vi "人脸检测.vi"(8 "错误输入（无错误）":errorcluster, 9 "face Parameter":T1, 10 "access_token":string, 11 "client_in":T2) -> (0 "错误输出":errorcluster, 2 "body":string caption="体部", 3 "client_out":T2)   [LabVIEW 2025, in "Baidu api.lvlib"]
uses:
  Baidu api.lvlib
  <vilib>/httpClient/ClientHandle.ctl
  <vilib>/httpClient/POSTBuffer.vi
  <vilib>/httpClient/LabVIEWHTTPClient.lvlib
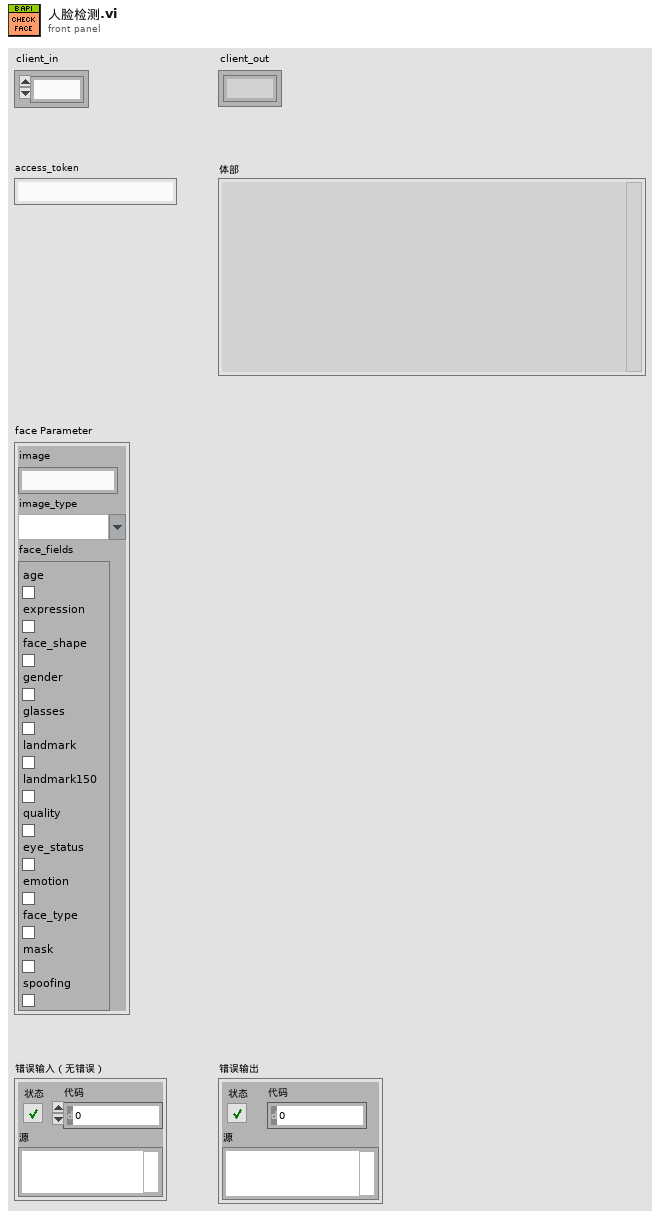
[diagram p1: front panel]
types:
  T1 = cluster{"image":string, "image_type":string, "face_fields ":cluster{"age":bool, "expression":bool, "face_shape":bool, "gender":bool, "glasses":bool, "landmark":bool, "landmark150":bool, "quality":bool, "eye_status":bool, "emotion":bool, "face_type":bool, "mask":bool, "spoofing":bool}}
  T2 = typedef "LabVIEWHTTPClient.lvlib/ClientHandle.ctl" = refnum<k1>
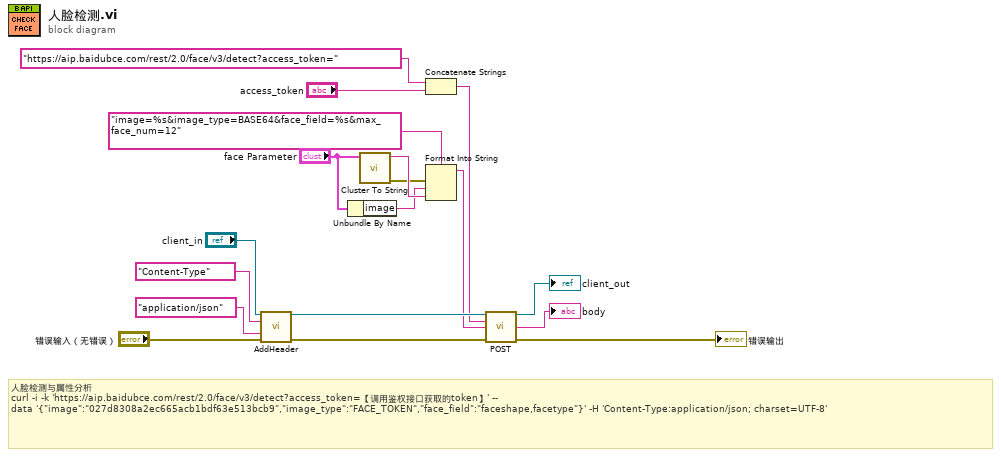
[diagram p0: block diagram]
diagram:
  # "人脸检测与属性分析\ncurl -i -k 'https://aip.baidubce.com/rest/2.0/face/v3/detect?access_token=【调用鉴权接口获取的token】' --\ndata '{\"image\":\"027d8308a2ec665acb1bdf63e513bcb9\",\"image_type\":\"FACE_TOKEN\",\"face_field\":\"faceshape,facetype\"}' -H 'Content-Type:application/json; charset=UTF-8'"
  n1 = call <vilib>:"AddHeader.vi"("client handle"="client_in", "header"="Content-Type", "value"="application/json", "error in (no error)"="错误输入（无错误）") -> ("client handle out"=w12:T2, "error out"=w16:errorcluster)  [unwired: 10 in]
  n2 = Unbundle By Name("face Parameter") -> ("image"=w2:string)
  n3 = call "Cluster To String.vi"("face Parameter"="face Parameter") -> ("error out"=w1:errorcluster, "String"=w4:string)  [unwired: 9 in]
  n4 = Concatenate Strings("https://aip.baidubce.com/rest/2.0/face/v3/detect?access_token=" ("url"), "access_token") -> (w10:string)
  n5 = Format Into String(format string="image=%s&image_type=BASE64&face_field=%s&max_face_num=12" ("格式字符串"), error in=w1, w2, w4) -> (resulting string=w5:string)  [unwired: 1 in, 1 out]
  n6 = call-poly <vilib>:"POST.vi"("client handle"=w12, "url"=w10, "buffer"=w5, "error in (no error)"=w16) -> ("client handle out"=→"client_out":T2, "body"=→"body":string, "error out"=→"错误输出":errorcluster)  [unwired: 8 in, 1 out]
